vi "Set ATM Message.vi"(8 "error in (no error)":errorcluster, 10 "Message Name":T1, 11 "ATM Controller in":refnum<class "ATM Controller.lvclass">) -> (0 "error out":errorcluster, 3 "ATM Controller out":refnum<class "ATM Controller.lvclass">)   [LabVIEW 2019, in "ATM Controller.lvlib" / "ATM Controller.lvclass"]
uses:
  ATM Controller.lvclass
  Message Name.ctl
  ATM Controller.lvclass/ATM Controller.ctl
  Simulated Display Console Actor/Simulated Display Console Actor Messages/Write Message Screen Msg/Write Message Screen Msg.lvclass/Write Message Screen Msg.ctl
  <vilib>/ActorFramework/Message Enqueuer/Message Enqueuer.lvclass/Message Enqueuer.ctl
  <vilib>/ActorFramework/Message Enqueuer/Enqueue.vi
  Simulated Display Console Actor/Simulated Display Console Actor Messages/Write Message Screen Msg/Write Message Screen Msg.lvclass
  C:/Program Files (x86)/National Instruments/LabVIEW 2019/vi.lib/ActorFramework/Message/Message.lvclass
  <vilib>/ActorFramework/Message Priority Queue/Priority Enqueue.vi
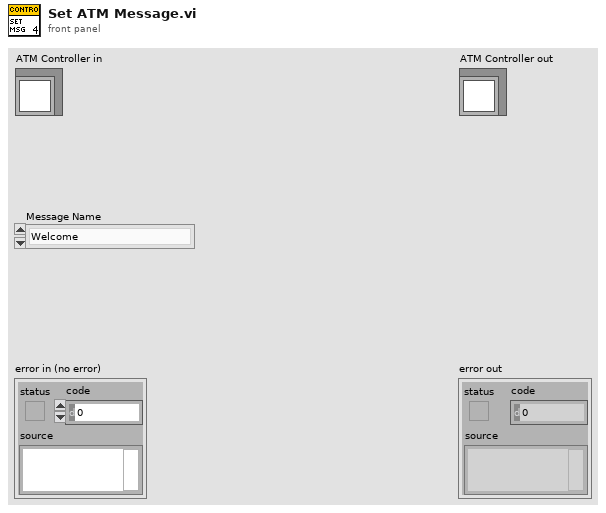
[diagram p1: front panel]
types:
  T1 = typedef "ATM Controller.lvlib/ATM Controller.lvclass/Message Name.ctl" = enum16{"Welcome", "Login", "Idle", "Invalid Login", "Terminate Session", "Deposit", "Withdrawal", "Fast Cash $50", "Withdrawal Failed", "Balance Inquiry"}
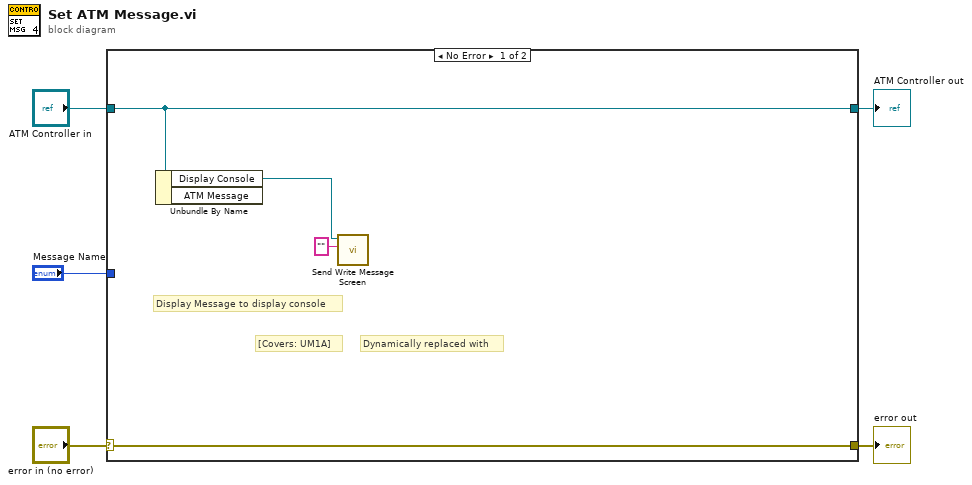
[diagram p0: block diagram]
diagram:
  n1 = case shown="No Error" "error in (no error)" {
    selector: "error in (no error)" -> [w9 w11]
    tunnel: [w9 w11] -> w4
    tunnel: [w8 w10] -> w2
    tunnel: "ATM Controller in" -> [w8 w10]
    tunnel: "Message Name" -> [_ _]
    frame No Error {
      # "Display Message to display console"
      # "Dynamically replaced with"
      # "[Covers: UM1A]"
      n2 = Unbundle By Name(w8) -> ("Display Console"=w6:refnum<class "Message Enqueuer.lvclass">)  [unwired: 1 out]
      n3 = call "Send Write Message Screen.vi"("Current Transaction"="", "Message Enqueuer"=w6) -> ()  [unwired: 8 in, 2 out]
    }
    frame Error {
    }
  }
  "error out" <- w4
  "ATM Controller out" <- w2
